vi "BIO_new_accept.vi"(8 "error in (no error)":errorcluster, 10 "Port (443)":string="443", 11 "SSL-Context in":refnum<class "SSL-Context.lvclass">) -> (0 "error out":errorcluster, 2 "Accept BIO out":refnum<class "BIO.lvclass">, 3 "SSL-Context out":refnum<class "SSL-Context.lvclass">)   [LabVIEW 2013, in "OpenSSL Socket.lvlib" / "SSL-Context.lvclass"]
uses:
  SSL-Context.lvclass
  BIO/BIO.lvclass
  SSL-Lib/SSL-Lib.lvclass/SSL-Lib.ctl
  BIO/BIO.lvclass/BIO.ctl
  SSL-Lib/Read Crypto Library Path.vi
  BIO/Write Handle.vi
  SSL-Lib/SSL-Lib.lvclass
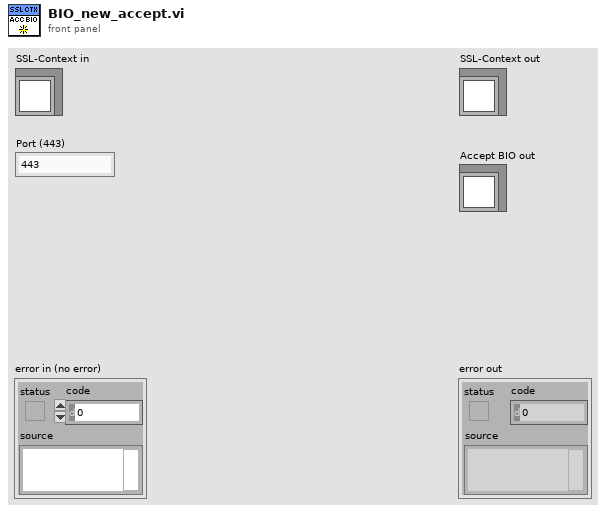
[diagram p1: front panel]
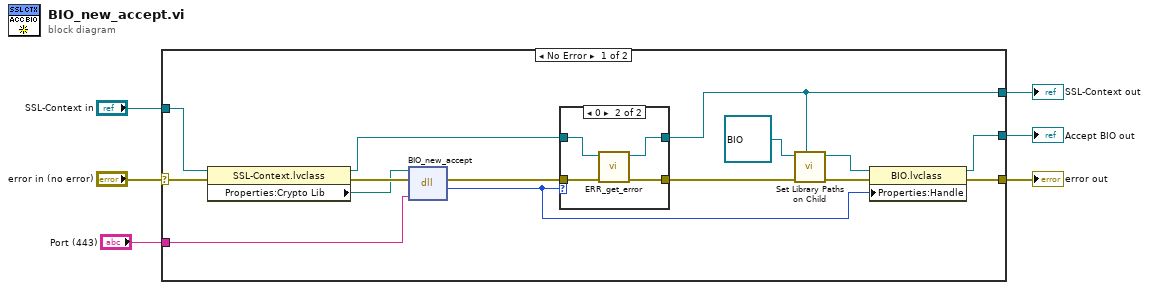
[diagram p0: block diagram]
diagram:
  n1 = case shown="No Error" "error in (no error)" {
    selector: "error in (no error)" -> [w21 w29]
    tunnel: [w14 w29] -> w5
    tunnel: [w10 w28] -> w3
    tunnel: "SSL-Context in" -> [w19 w28]
    tunnel: [w13 _] -> w2
    tunnel: "Port (443)" -> [w7 _]
    frame No Error {
      n2 = property class="SSL-Context.lvclass"(reference=w19, error in=w21) -> (reference out=w11:refnum<class "SSL-Context.lvclass">, error out=w20:errorcluster, "Properties:Crypto Lib"=w18:path)
      n3 = dll-call lib="C:/Program Files (x86)/National Instruments/Shared/nissl/NIlibeay32.dll" fn="BIO_new_accept"(path in=w18, error in=w20, "host_port"=w7) -> (error out=w12:errorcluster, "return type"=w8:u64)  [unwired: 2 in, 1 out]
      n4 = case shown="0" w8 {
        tunnel: w12 -> [w23 w27]
        tunnel: w11 -> [w22 w26]
        tunnel: [w22 w25] -> w10
        tunnel: [w23 w24] -> w9
        frame Default {
        }
        frame 0 {
          n5 = call "ERR_get_error.vi"("error in (no error)"=w27, "SSL-Lib in"=w26) -> ("error out"=w24:errorcluster, "SSL-Lib out"=w25:refnum<class "SSL-Context.lvclass">)  [unwired: 8 in]
        }
      }
      n6 = call-dynamic "Set Library Paths on Child.vi"(7:"SSL-Lib in"=w10, "error in (no error)"=w9, 11:"SSL-Lib in"=refnum<class "BIO.lvclass"> refnum ("SSL_Lib.lvlib:BIO.lvclass")) -> ("error out"=w16:errorcluster, "SSL-Lib out"=w15:refnum<class "BIO.lvclass">)  [unwired: 7 in]
      n7 = property class="BIO.lvclass"(reference=w15, error in=w16, "Properties:Handle"=w8) -> (reference out=w13:refnum<class "BIO.lvclass">, error out=w14:errorcluster)
    }
    frame Error {
    }
  }
  "error out" <- w5
  "SSL-Context out" <- w3
  "Accept BIO out" <- w2
